vi "Sweep Pulsemode.vi"(7 "Pulse Mode (F: Disabled)":bool, 8 "error in":errorcluster, 9 "Channel (Channel A)":T1, 10 "Node In":string, 11 "VISA resource name":refnum<visa-resource-name>) -> (0 "error out":errorcluster, 2 "Node Out":string, 3 "VISA resource name out":refnum<visa-resource-name>, 4 "Command String":string)   [LabVIEW 2018, in "Keithley 2600 Series.lvlib"]
doc: "This VI sets the pulsemode for the sweep.\n\nSet pulse mode to disabled for traditional sweeps.\n\n<b>Functions and Attributes Used</b>\nsmuX.trigger.endpulse.action"
uses:
  Keithley 2600 Series.lvlib
  Private/GlobalVariables.vi
  Channel.ctl
panel:
  # "(c) 2008 Keithley Instruments, Inc.  ALL RIGHTS RESERVED."
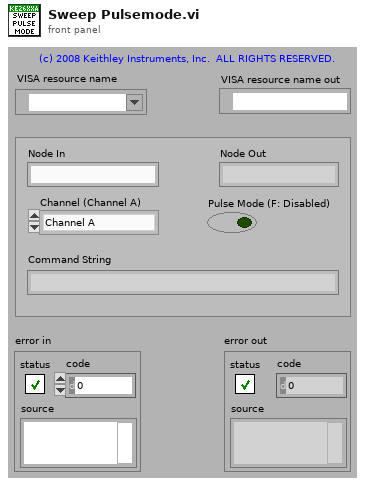
[diagram p1: front panel]
types:
  T1 = typedef "Keithley 2600 Series.lvlib/Channel.ctl" = enum32{"Channel A", "Channel B"}
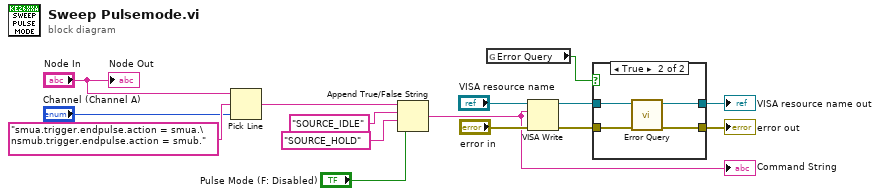
[diagram p0: block diagram]
diagram:
  n1 = Pick Line(string ("")="Node In", multi-line string="smua.trigger.endpulse.action = smua.\nsmub.trigger.endpulse.action = smub.", line index="Channel (Channel A)") -> (output string=w5:string)
  n2 = Append True/False String(1:"Pulse Mode (F: Disabled)", 2:"SOURCE_HOLD" ("multi-line string"), 3:"SOURCE_IDLE" ("true string"), 4:w5) -> (0:w4:string)
  "Command String" <- w4
  n3 = global read "GlobalVariables.vi" "Error Query"() -> (w10:bool)
  n4 = VISA Write(VISA resource name="VISA resource name", write buffer=w4, error in (no error)="error in") -> (VISA resource name out=w9:refnum<visa-resource-name>, error out=w8:errorcluster)  [unwired: 1 out]
  n5 = case shown="True" w10 {
    tunnel: w9 -> [w17 w21]
    tunnel: w8 -> [w16 w20]
    tunnel: [w17 w19] -> w7
    tunnel: [w16 w18] -> w6
    frame False {
    }
    frame True {
      n6 = call "Error Query.vi"("error in (no error)"=w20, "VISA resource name"=w21) -> ("error out"=w18:errorcluster, "VISA resource name out"=w19:refnum<visa-resource-name>)  [unwired: 8 out]
    }
  }
  "VISA resource name out" <- w7
  "error out" <- w6
  "Node Out" <- "Node In"
